vi "DSF.Engine.Framework.Create.Transfers.vi"(8 "error in (no error)":errorcluster, 10 "Transfer Configurations":refnum<class "DSF.Shared.Configuration.Transfer.lvclass">[](array[class]), 11 "Framework in":refnum<class "DSF.Engine.Framework.lvclass">) -> (0 "error out":errorcluster, 2 "Transfers":refnum<class "DSF.Engine.Transfer.lvclass">[](array[class]), 3 "Framework out":refnum<class "DSF.Engine.Framework.lvclass">)   [LabVIEW 2017, in "DSF.Engine.lvlib" / "DSF.Engine.Framework.lvclass"]
uses:
  DSF.Engine.Framework.lvclass
  Transfer/DSF.Engine.Transfer.lvclass
  Shared/Classes/Transfer/DSF.Shared.Configuration.Transfer.lvclass
  DSF.Engine.Framework.lvclass/DSF.Engine.Framework.ctl
  Cache/DSF.Engine.Memory.Cache.lvclass/DSF.Engine.Memory.Cache.ctl
  Shared/Classes/Transfer/DSF.Shared.Configuration.Transfer.lvclass/DSF.Shared.Configuration.Transfer.ctl
  <vilib>/National Instruments/Memory Manager/Classes/Pointer/Memory.Pointer.lvclass/Memory.Pointer.ctl
  <vilib>/National Instruments/Memory Manager/Classes/Pointer/Memory.Pointer.Get Size.vi
  <vilib>/National Instruments/Memory Manager/Classes/Pointer/Memory.Pointer.Allocate.vi
  <vilib>/National Instruments/Memory Manager/Classes/Pointer/Memory.Pointer.Copy All.vi
  <vilib>/National Instruments/Memory Manager/Classes/Pointer/Memory.Pointer.Set Address.vi
  <vilib>/National Instruments/Memory Manager/Classes/Pointer/Memory.Pointer.Set Size.vi
  <vilib>/National Instruments/Memory Manager/Classes/Pointer/Memory.Pointer.Set Allocated.vi
  <vilib>/National Instruments/Memory Manager/Classes/Pointer/Memory.Pointer.Copy.vi
  <vilib>/National Instruments/Memory Manager/Classes/Pointer/Memory.Pointer.Copy.No Check.vi
  <vilib>/National Instruments/Memory Manager/Classes/Pointer/Memory.Pointer.Parameter Check.Subset.vi
  <vilib>/National Instruments/Memory Manager/Classes/Pointer/Memory.Pointer.Parameter Check.Null Pointer.vi
  <vilib>/National Instruments/Memory Manager/Classes/Pointer/Memory.Pointer.Get Address.vi
  <vilib>/National Instruments/Memory Manager/Classes/Pointer/Memory.Pointer.Errors.vi
  <vilib>/National Instruments/Memory Manager/Classes/Pointer/Memory.Pointer.Errors.Out of Bounds.vi
  <vilib>/National Instruments/Memory Manager/Classes/Pointer/Memory.Pointer.Errors.Null Pointer.vi
  <vilib>/NI/Static Error Handling/VIs/Static Error Handling.Source Buffer.Write.String.vi
  <vilib>/National Instruments/Memory Manager/Classes/Pointer/Memory.Pointer.Errors.Write Pointer Size.vi
  <vilib>/National Instruments/Memory Manager/Classes/Pointer/Memory.Pointer.Errors.Create Error.vi
  <vilib>/NI/Static Error Handling/VIs/Static Error Handling.Source Buffer.Write.Numeric.Scalar.Base10.vi
  <vilib>/NI/Static Error Handling/VIs/Static Error Handling.Source Buffer.Write.Numeric.Scalar.Base10 (U64).vi
  <vilib>/NI/Static Error Handling/VIs/Static Error Handling.Error Cluster Constant.vi
  <vilib>/NI/Static Error Handling/VIs/Static Error Handling.Error Cluster Constant (512B).vi
  <vilib>/NI/Static Error Handling/VIs/Static Error Handling.Parameters.Status.Set.vi
  <vilib>/NI/Static Error Handling/VIs/Static Error Handling.Parameters.Code.Set.vi
  <vilib>/NI/Static Error Handling/VIs/Static Error Handling.Parameters.VI Source.Set.vi
  <vilib>/National Instruments/Memory Manager/Constants/Memory.Constants.vi
  <vilib>/National Instruments/Memory Manager/Constants/Memory.Constants.Library Name.vi
  <vilib>/National Instruments/Memory Manager/Classes/Pointer/Memory.Pointer.Errors.Get Info.vi
  Pointer/DSF.Engine.Pointer.DBL.lvclass
  C:/Program Files (x86)/National Instruments/LabVIEW 2017/vi.lib/National Instruments/Memory Manager/Classes/Pointer/Memory.Pointer.lvclass
  <vilib>/National Instruments/Memory Manager/Classes/Pointer/Memory.Pointer.lvclass
  Buffer/DSF.Engine.Memory.Buffer.lvclass
  Cache/DSF.Engine.Memory.Cache.lvclass
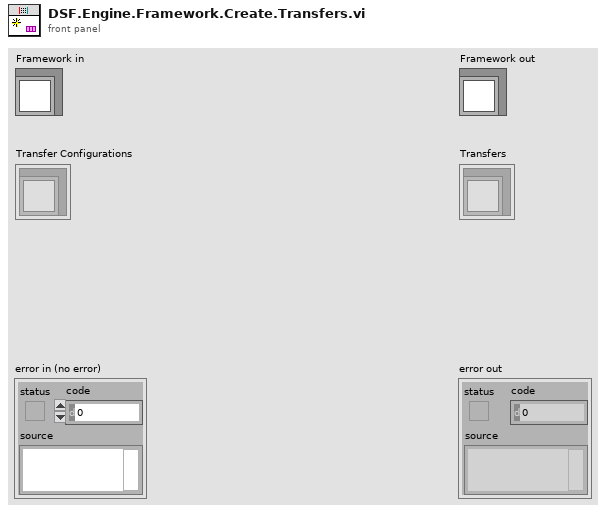
[diagram p1: front panel]
types:
  T1 = typedef "DSF.Shared.lvlib/DSF.Shared.Refactor.Typedefs.Channel Block.ctl" = cluster{"data type":T2, "count":u64, "buffer offset":u64}
  T2 = typedef "DSF.Shared.lvlib/DSF.Shared.Typedefs.Data Type.ctl" = enum8{"Bool", "SGL", "DBL", "I8", "I16", "I32", "I64", "U8", "U16", "U32", "U64"}
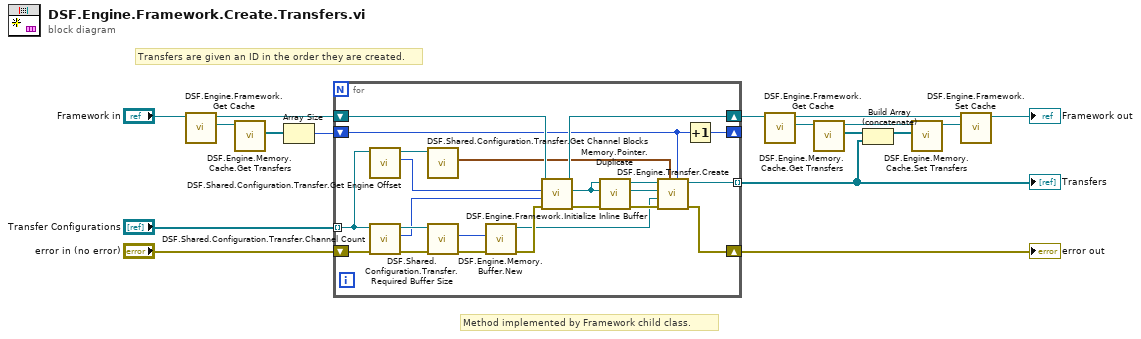
[diagram p0: block diagram]
diagram:
  # "Method implemented by Framework child class."
  # "Transfers are given an ID in the order they are created."
  n1 = call "DSF.Engine.Framework.Get Cache.vi"("Framework in"="Framework in") -> ("Cache"=w10:refnum<class "DSF.Engine.Memory.Cache.lvclass">, "Framework out"=w11:refnum<class "DSF.Engine.Framework.lvclass">)  [unwired: 9 in]
  n2 = call "DSF.Engine.Memory.Cache.Get Transfers.vi"("Cache in"=w10) -> ("Transfers"=w13:refnum<class "DSF.Engine.Transfer.lvclass">[])  [unwired: 9 in, 1 out]
  n3 = Array Size(array=w13) -> (size(s)=w14:i32)
  n4 = for {
    shift-right: [w40] -> w17
    shift-left: "error in (no error)" -> [w23]
    tunnel: [w39] -> w6 mode=indexing
    shift-right: [w28] -> w8
    shift-left: w11 -> [w38]
    tunnel: "Transfer Configurations" -> [w36] mode=indexing
    shift-right: [w21] -> _
    shift-left: w14 -> [w20]
    n5 = call "DSF.Shared.Configuration.Transfer.Get Engine Offset.vi"("Transfer Configuration in"=w36) -> ("engine offset"=w37:u64, "Transfer Configuration out"=w19:refnum<class "DSF.Shared.Configuration.Transfer.lvclass">)  [unwired: 9 in]
    n6 = call "DSF.Shared.Configuration.Transfer.Channel Count.vi"("error in (no error)"=w23, "Transfer Configuration in"=w36) -> ("error out"=w24:errorcluster, "total channel count"=w29:u64, "Transfer Configuration out"=w30:refnum<class "DSF.Shared.Configuration.Transfer.lvclass">)  [unwired: 7 in]
    n7 = call "DSF.Shared.Configuration.Transfer.Get Channel Blocks.vi"("Transfer Configuration in"=w19) -> ("channel blocks"=w18:T1[])  [unwired: 9 in, 1 out]
    n8 = call "DSF.Shared.Configuration.Transfer.Required Buffer Size.vi"("error in (no error)"=w24, "Transfer Configuration in"=w30) -> ("error out"=w22:errorcluster, "required buffer size"=w26:u64)  [unwired: 7 in, 1 out]
    n9 = call "DSF.Engine.Memory.Buffer.New.vi"("error in (no error)"=w22, "size"=w26) -> ("error out"=w27:errorcluster, "Buffer out"=w25:refnum<class "DSF.Engine.Memory.Buffer.lvclass">)  [unwired: 8 in]
    n10 = call-dynamic "DSF.Engine.Framework.Initialize Inline Buffer.vi"("error in (no error)"=w27, "channel count"=w29, "first channel offset"=w37, "Framework in"=w38) -> ("error out"=w31:errorcluster, "Buffer"=w32:refnum<class "DSF.Engine.Pointer.DBL.lvclass">, "Framework out"=w28:refnum<class "DSF.Engine.Framework.lvclass">)  [unwired: 5 in]
    n11 = call <vilib>:"Memory.Pointer.Duplicate.vi"("error in (no error)"=w31, "new Pointer type"=w32, "Pointer in"=w32) -> ("error out"=w35:errorcluster, "new duplicate Pointer"=w34:refnum<class "DSF.Engine.Pointer.DBL.lvclass">, "Pointer out"=w33:refnum<class "DSF.Engine.Pointer.DBL.lvclass">)  [unwired: 6 in]
    n12 = call "DSF.Engine.Transfer.Create.vi"("id"=w20, "channel blocks"=w18, "error in (no error)"=w35, "String Buffer"=w25, "Intermediate Buffer"=w34, "Inline Buffer"=w33) -> ("error out"=w40:errorcluster, "Transfer out"=w39:refnum<class "DSF.Engine.Transfer.lvclass">)  [unwired: 4 in]
    n13 = Increment(x=w20) -> (x+1=w21:i32)
  }
  "error out" <- w17
  "Transfers" <- w6
  n14 = call "DSF.Engine.Framework.Get Cache.vi"("Framework in"=w8) -> ("Cache"=w9:refnum<class "DSF.Engine.Memory.Cache.lvclass">, "Framework out"=w5:refnum<class "DSF.Engine.Framework.lvclass">)  [unwired: 9 in]
  n15 = call "DSF.Engine.Memory.Cache.Get Transfers.vi"("Cache in"=w9) -> ("Transfers"=w7:refnum<class "DSF.Engine.Transfer.lvclass">[], "Cache out"=w1:refnum<class "DSF.Engine.Memory.Cache.lvclass">)  [unwired: 9 in]
  n16 = Build Array (concatenate)(w7, w6) -> (w4:refnum<class "DSF.Engine.Transfer.lvclass">[])
  n17 = call "DSF.Engine.Memory.Cache.Set Transfers.vi"("Transfers"=w4, "Cache in"=w1) -> ("Cache out"=w3:refnum<class "DSF.Engine.Memory.Cache.lvclass">)  [unwired: 9 in]
  n18 = call "DSF.Engine.Framework.Set Cache.vi"("Cache"=w3, "Framework in"=w5) -> ("Framework out"=→"Framework out":refnum<class "DSF.Engine.Framework.lvclass">)  [unwired: 9 in]
